vi "Grafica all plots.vi"(0 "prova":i32, 1 "ID COLLEGAMENTI":i32[](array[numeric]), 2 "Array scelte grafici":refnum<vi>[](array[refnum]), 3 "Array Grafici":refnum<vi>[](array[refnum]), 4 "array interpolazioni":refnum<vi>[](array[refnum]), 5 "Collaudi di confronto":T3[](array[typedef]), 6 "Array plot":T2[](array[typedef]) {"PLOT"."GRANDEZZA Y" items=["Banco", "Anno", "Numero", "N° tabella", "Misura", "Tipo prova", "Progressivo Acq", "tempo[h:m:s]", "tempo acq[min]", "f [Hz]", "Uav [V]", "Iav [A]", "Tq [Nm]", "n [rpm]", "P1 [kW]", "P1 n[kW]", "Q [m3/h]", "Q n[m3/h]", "Q [l/min]", "Q n[l/min]", "H1 [m]", "Dislivello [m]", "Hdinamica [m]", "HvAsp [m]", "HvMand [m]", "HvTot [m]", "H2 [m]", "Htot [m]", "Htot n[m]", "P3 (Phyd) [kW]", "P3 (Phyd) n[kW]", "P2 [kW]", "P2 n[kW]", "P2 n ps[kW]", "eta motore [%]", "eta pompa [%]", "eta pompa n[%]", "eta gruppo [%]", "eta gruppo n[%]", "T acqua [°C]", "Densità liquido [kg/m3]", "P barometrica [mbar]", "pf", "Uch1 [V]", "Uch2 [V]", "Uch3 [V]", "Ich1 [A]", "Ich2 [A]", "Ich3 [A]", "Temp.amb[°C]", "Ru-w [ohm]", "DTavvolg. [°C]", "Tamb Freddo [°C]", "Ru-w Freddo [ohm]", "Tc1[°C]", "Tc2[°C]", "Tc3[°C]", "Tc4[°C]", "Tc5", "Tc6", "Tc7", "Tc8", "H1[Bar]", "H2[bar]", "P premist.[Bar]", "Pserb[bar]", "n°NPSH", "NPSH", "Htot Ref[m]", "NPSH_%caduta", "%caduta", "Qref [m3/h]", "MEI"]; "PLOT"."GRANDEZZA X" items=["Banco", "Anno", "Numero", "N° tabella", "Misura", "Tipo prova", "Progressivo Acq", "tempo[h:m:s]", "tempo acq[min]", "f [Hz]", "Uav [V]", "Iav [A]", "Tq [Nm]", "n [rpm]", "P1 [kW]", "P1 n[kW]", "Q [m3/h]", "Q n[m3/h]", "Q [l/min]", "Q n[l/min]", "H1 [m]", "Dislivello [m]", "Hdinamica [m]", "HvAsp [m]", "HvMand [m]", "HvTot [m]", "H2 [m]", "Htot [m]", "Htot n[m]", "P3 (Phyd) [kW]", "P3 (Phyd) n[kW]", "P2 [kW]", "P2 n[kW]", "P2 n ps[kW]", "eta motore [%]", "eta pompa [%]", "eta pompa n[%]", "eta gruppo [%]", "eta gruppo n[%]", "T acqua [°C]", "Densità liquido [kg/m3]", "P barometrica [mbar]", "pf", "Uch1 [V]", "Uch2 [V]", "Uch3 [V]", "Ich1 [A]", "Ich2 [A]", "Ich3 [A]", "Temp.amb[°C]", "Ru-w [ohm]", "DTavvolg. [°C]", "Tamb Freddo [°C]", "Ru-w Freddo [ohm]", "Tc1[°C]", "Tc2[°C]", "Tc3[°C]", "Tc4[°C]", "Tc5", "Tc6", "Tc7", "Tc8", "H1[Bar]", "H2[bar]", "P premist.[Bar]", "Pserb[bar]", "n°NPSH", "NPSH", "Htot Ref[m]", "NPSH_%caduta", "%caduta", "Qref [m3/h]", "MEI"]; "Assi grafico"."ASSE X" items=["X 1", "X 2"]; "Assi grafico"."ASSE Y" items=["Y 1", "Y 2", "Y 3", "Y 4"]}, 7 "Dati collaudo in corso":T3, 8 "Tabella in corso":i32, 9 "grafico generico":cluster{"X":i32, "Y":i32, "nome plot":string}, 10 "Grafici":T1[](array[typedef]) {"ASSE Y 5"."Decimali" min=0 max=6; "ASSE Y 4"."Decimali" min=0 max=6; "ASSE Y 3"."Decimali" min=0 max=6; "ASSE Y 2"."Decimali" min=0 max=6; "ASSE Y 1"."Decimali" min=0 max=6; "ASSE X 2"."Decimali" min=0 max=6; "ASSE X 1"."Decimali" min=0 max=6}, 11 "Legend:Autosize":bool) -> ()   [LabVIEW 2019]
uses:
  TypeDef/Dati collaudo.ctl
  TypeDef/Definizione_plot.ctl
  TypeDef/Definizione_Grafico_REPORT.ctl
panel:
  out "Array AND":bool[](array[boolean])
  out "Array Prova Resistenza":bool[](array[boolean])
  out "Nomi Grafici":string[](array[string])
  out "x-y":u32
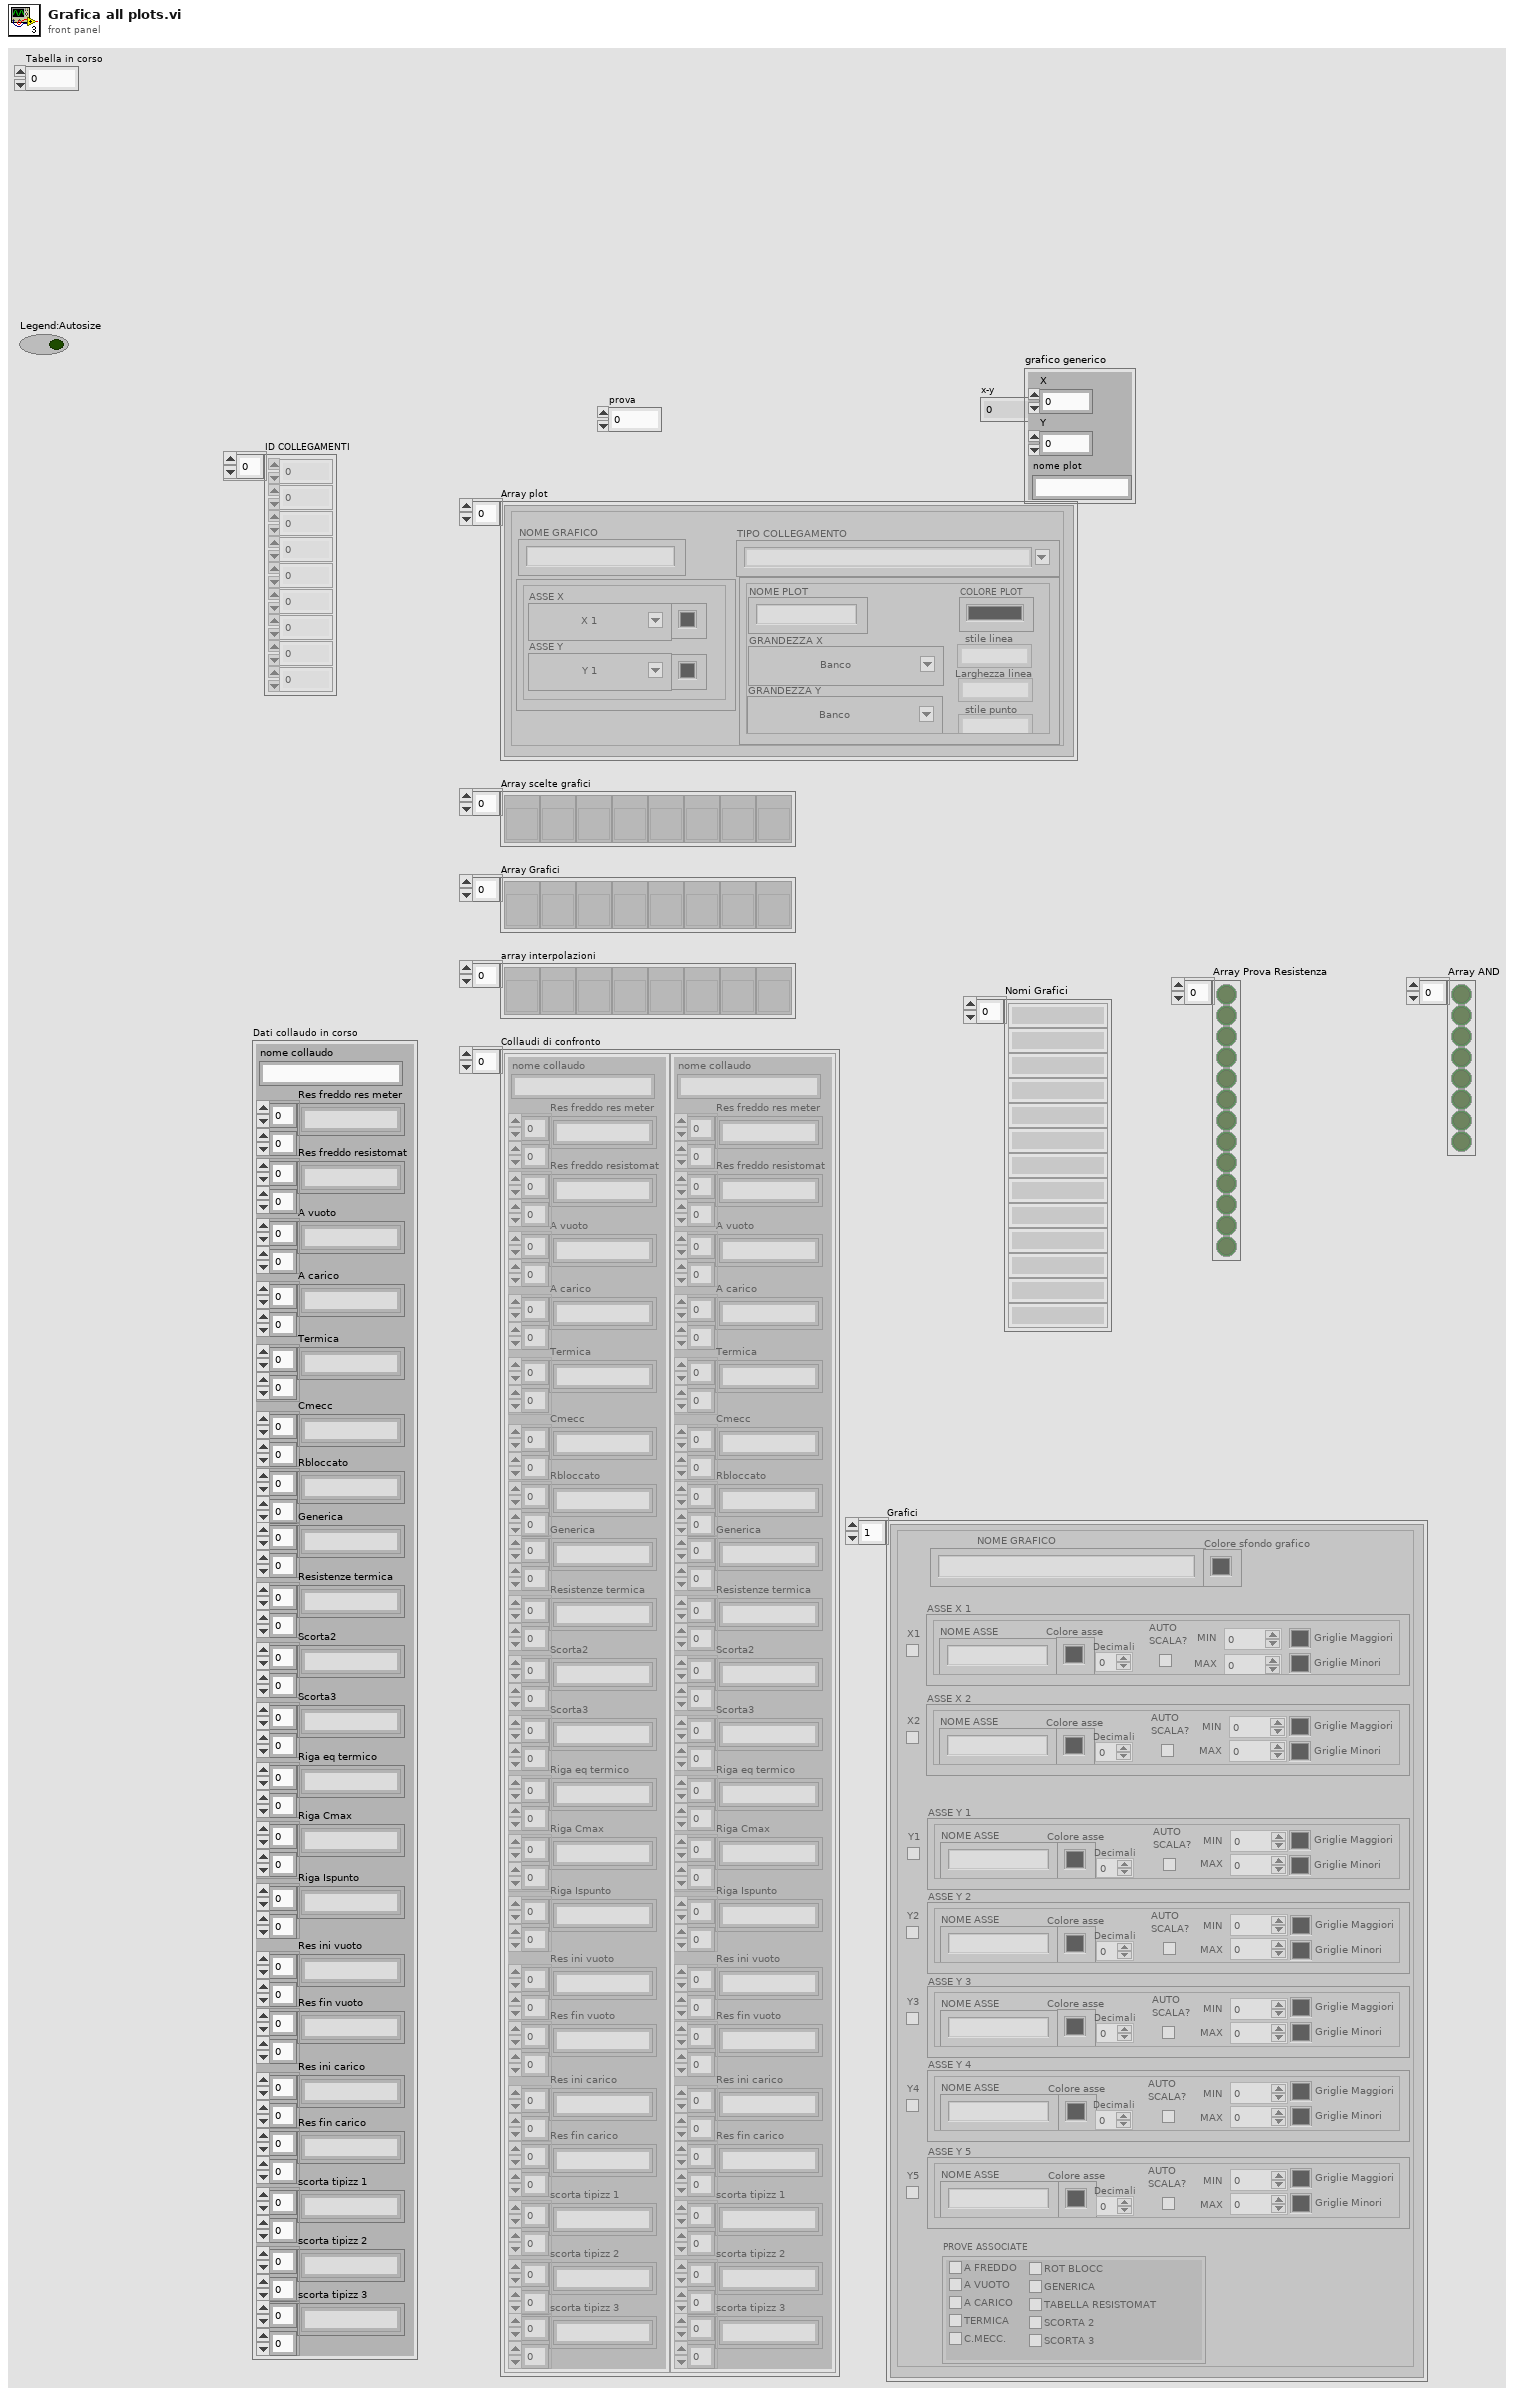
[diagram p1: front panel]
types:
  T1 = typedef "Definizione_Grafico_REPORT.ctl" = cluster{"ASSE X 1":cluster{"NOME ASSE":string, "AUTO\nSCALA?":bool, "MIN":dbl, "MAX":dbl, "Colore asse":u32, "Griglie Maggiori":u32, "Griglie Minori":u32, "Decimali":i8}, "ASSE X 2":cluster{"NOME ASSE":string, "AUTO\nSCALA?":bool, "MIN":dbl, "MAX":dbl, "Colore asse":u32, "Griglie Maggiori":u32, "Griglie Minori":u32, "Decimali":i8}, "ASSE Y 1":cluster{"NOME ASSE":string, "AUTO\nSCALA?":bool, "MIN":dbl, "MAX":dbl, "Colore asse":u32, "Griglie Maggiori":u32, "Griglie Minori":u32, "Decimali":i8}, "ASSE Y 2":cluster{"NOME ASSE":string, "AUTO\nSCALA?":bool, "MIN":dbl, "MAX":dbl, "Colore asse":u32, "Griglie Maggiori":u32, "Griglie Minori":u32, "Decimali":i8}, "ASSE Y 3":cluster{"NOME ASSE":string, "AUTO\nSCALA?":bool, "MIN":dbl, "MAX":dbl, "Colore asse":u32, "Griglie Maggiori":u32, "Griglie Minori":u32, "Decimali":i8}, "ASSE Y 4":cluster{"NOME ASSE":string, "AUTO\nSCALA?":bool, "MIN":dbl, "MAX":dbl, "Colore asse":u32, "Griglie Maggiori":u32, "Griglie Minori":u32, "Decimali":i8}, "X1":bool, "X2":bool, "Y1":bool, "Y2":bool, "Y3":bool, "Y4":bool, "NOME GRAFICO":string, "PROVE ASSOCIATE":cluster{"A FREDDO":bool, "A VUOTO":bool, "A CARICO":bool, "TERMICA":bool, "C.MECC.":bool, "ROT BLOCC":bool, "GENERICA":bool, "TABELLA RESISTOMAT":bool, "SCORTA 2":bool, "SCORTA 3":bool}, "ASSE Y 5":cluster{"NOME ASSE":string, "AUTO\nSCALA?":bool, "MIN":dbl, "MAX":dbl, "Colore asse":u32, "Griglie Maggiori":u32, "Griglie Minori":u32, "Decimali":i8}, "Y5":bool, "Colore sfondo grafico":u32}
  T2 = typedef "Definizione_plot.ctl" = cluster{"Assi grafico":cluster{"ASSE Y":u16, "ASSE X":u16, "Colore x":u32, "Colore y":u32}, "TIPO COLLEGAMENTO":string, "PLOT":cluster{"GRANDEZZA X":u16, "GRANDEZZA Y":u16, "COLORE PLOT":u32, "NOME PLOT":string, "Larghezza linea":u16, "stile linea":u16, "stile punto":u16}, "NOME GRAFICO":string}
  T3 = typedef "Dati collaudo.ctl" = cluster{"nome collaudo":string, "Res freddo res meter":string[][], "Res freddo resistomat":string[][], "A vuoto":string[][], "A carico":string[][], "Termica":string[][], "Cmecc":string[][], "Rbloccato":string[][], "Generica":string[][], "Resistenze termica":string[][], "Scorta2":string[][], "Scorta3":string[][], "Riga eq termico":string[][], "Riga Cmax":string[][], "Riga Ispunto":string[][], "Res ini vuoto":string[][], "Res fin vuoto":string[][], "Res ini carico":string[][], "Res fin carico":string[][], "scorta tipizz 1":string[][], "scorta tipizz 2":string[][], "scorta tipizz 3":string[][]}
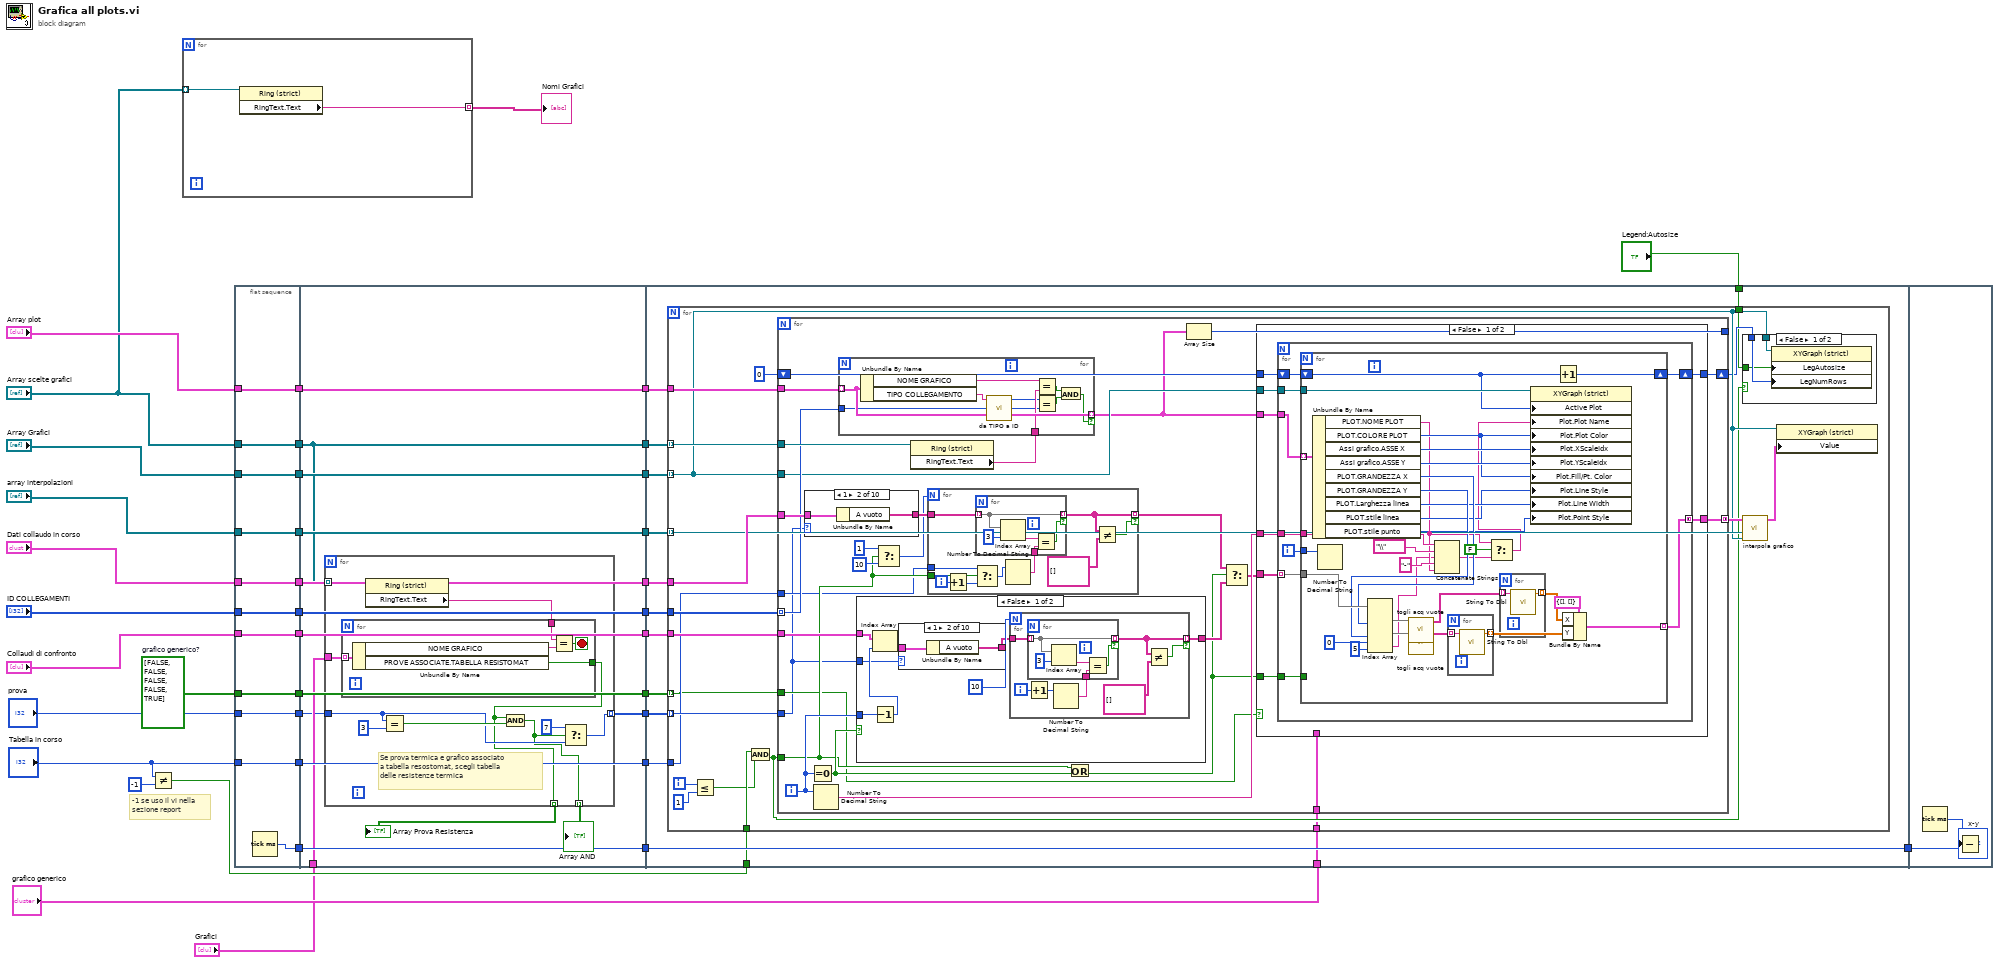
[diagram p0: block diagram]
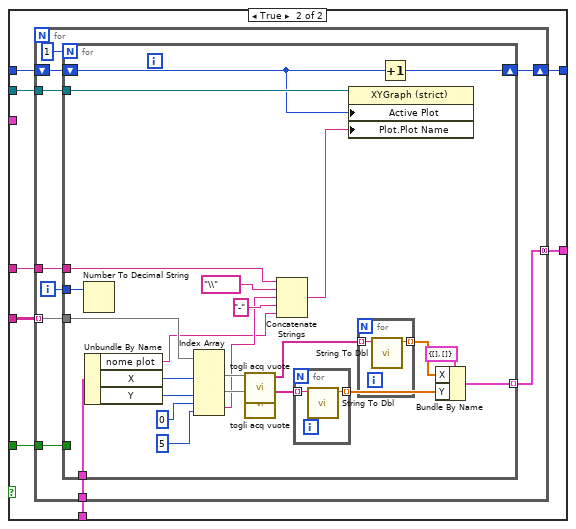
[diagram p3: hidden frame]
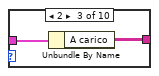
[diagram p5: hidden frame]
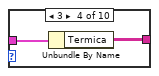
[diagram p6: hidden frame]
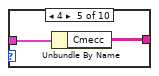
[diagram p7: hidden frame]
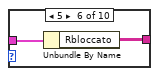
[diagram p8: hidden frame]
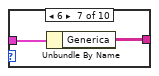
[diagram p9: hidden frame]
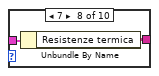
[diagram p10: hidden frame]
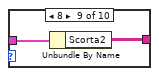
[diagram p11: hidden frame]
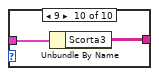
[diagram p12: hidden frame]
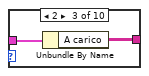
[diagram p14: hidden frame]
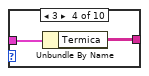
[diagram p15: hidden frame]
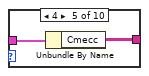
[diagram p16: hidden frame]
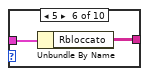
[diagram p17: hidden frame]
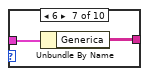
[diagram p18: hidden frame]
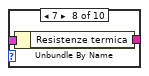
[diagram p19: hidden frame]
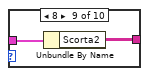
[diagram p20: hidden frame]
diagram:
  w6 = bool[] [FALSE, FALSE, FALSE, FALSE, TRUE]  # grafico generico?
  # "-1 se uso il vi nella\nsezione report"
  n1 = Not Equal?(x="Tabella in corso", y=-1) -> (x != y?=w29:bool)
  n2 = for {
    tunnel: "Array scelte grafici" -> [w41] mode=indexing
    tunnel: [w40] -> w2 mode=indexing
    n3 = property class="Ring (strict)"(reference=w41) -> ("RingText.Text"=w40:string)  [unwired: 1 in, 2 out]
  }
  "Nomi Grafici" <- w2
  n4 = flat-sequence {
    tunnel: "prova" -> [w45]
    tunnel: "Array scelte grafici" -> [w46]
    tunnel: "Array Grafici" -> [w47]
    tunnel: "Array plot" -> [w48]
    tunnel: "Dati collaudo in corso" -> [w49]
    tunnel: "Collaudi di confronto" -> [w50]
    tunnel: "ID COLLEGAMENTI" -> [w51]
    tunnel: "array interpolazioni" -> [w52]
    tunnel: [w52] -> w28
    tunnel: [w51] -> w26
    tunnel: [w50] -> w24
    tunnel: [w49] -> w22
    tunnel: [w48] -> w20
    tunnel: [w47] -> w18
    tunnel: [w46] -> w16
    tunnel: [w45] -> w14
    tunnel: [w44] -> w12
    tunnel: "Tabella in corso" -> [w43]
    tunnel: [w43] -> w10
    tunnel: [w42] -> w7
    tunnel: w6 -> [w42]
    tunnel: w28 -> [w67]
    tunnel: [w67] -> w27
    tunnel: w26 -> [w66]
    tunnel: [w66] -> w25
    tunnel: w24 -> [w65]
    tunnel: [w65] -> w23
    tunnel: w22 -> [w64]
    tunnel: [w64] -> w21
    tunnel: w20 -> [w63]
    tunnel: [w63] -> w19
    tunnel: w18 -> [w60]
    tunnel: [w60] -> w17
    tunnel: w16 -> [w57]
    tunnel: [w57] -> w15
    tunnel: w14 -> [w56]
    tunnel: [w55] -> w13
    tunnel: w12 -> [w62]
    tunnel: [w62] -> w11
    tunnel: w10 -> [w61]
    tunnel: [w61] -> w9
    tunnel: [w59] -> w8
    tunnel: w7 -> [w59]
    tunnel: "Grafici" -> [w58]
    tunnel: w27 -> [w96]
    tunnel: w25 -> [w95]
    tunnel: w23 -> [w94]
    tunnel: w21 -> [w93]
    tunnel: w19 -> [w92]
    tunnel: w17 -> [w91]
    tunnel: w15 -> [w90]
    tunnel: w13 -> [w89]
    tunnel: w11 -> [w88]
    tunnel: [w88] -> w32
    tunnel: w9 -> [w87]
    tunnel: w29 -> [w86]
    tunnel: w8 -> [w85]
    tunnel: "grafico generico" -> [w84]
    tunnel: "Legend:Autosize" -> [w83]
    tunnel: w32 -> [w329]
    frame #0 {
      n5 = Tick Count (ms)() -> (millisecond timer value=w44:u32)
    }
    frame #1 {
      n6 = for {
        tunnel: w58 -> [w77]
        tunnel: w57 -> [w76] mode=indexing
        tunnel: w56 -> [w72]
        tunnel: [w71] -> w55 mode=indexing
        tunnel: [w69] -> w54 mode=indexing
        tunnel: [w68] -> w53 mode=indexing
        # "Se prova termica e grafico associato\na tabella resostomat, scegli tabella \ndelle resistenze termica"
        n7 = property class="Ring (strict)"(reference=w76) -> ("RingText.Text"=w75:string)  [unwired: 1 in, 2 out]
        n8 = for {
          tunnel: w77 -> [w82] mode=indexing
          tunnel: w75 -> [w80]
          tunnel: [w78] -> w69
          stop <- w79 stop-if-true
          n9 = Unbundle By Name(w82) -> ("NOME GRAFICO"=w81:string, "PROVE ASSOCIATE.TABELLA RESISTOMAT"=w78:bool)
          n10 = Equal?(x=w80, y=w81) -> (x = y?=w79:bool)
        }
        n11 = Equal?(x=w72, y=3) -> (x = y?=w73:bool)
        n12 = And(x=w69, y=w73) -> (x .and. y?=w68:bool)
        n13 = Select(t=7, s=w68, f=w72) -> (s? t:f=w71:i32)
      }
      "Array Prova Resistenza" <- w54
      "Array AND" <- w53
    }
    frame #2 {
      n14 = for {
        tunnel: w90 -> [w113] mode=indexing
        tunnel: w91 -> [w107] mode=indexing
        tunnel: w92 -> [w117]
        tunnel: w93 -> [w116]
        tunnel: w94 -> [w115]
        tunnel: w95 -> [w114]
        tunnel: w96 -> [w110] mode=indexing
        tunnel: w89 -> [w109] mode=indexing
        tunnel: w87 -> [w104]
        tunnel: w86 -> [w103]
        tunnel: w85 -> [w99] mode=indexing
        tunnel: w84 -> [w98]
        tunnel: w83 -> [w97]
        i -> [w106]
        n15 = Less Or Equal?(x=w106, y=1) -> (x <= y?=w102:bool)
        n16 = And(x=w103, y=w102) -> (x .and. y?=w101:bool)
        n17 = for {
          tunnel: w117 -> [w147]
          tunnel: w113 -> [w146]
          tunnel: w107 -> [w141]
          tunnel: w116 -> [w145]
          tunnel: w115 -> [w135]
          tunnel: w114 -> [w144] mode=indexing
          tunnel: [w140] -> w112 mode=concatenating
          shift-right: [w139] -> w100
          shift-left: 0 -> [w138]
          tunnel: w109 -> [w121]
          tunnel: [w130] -> _
          tunnel: w101 -> [w126]
          tunnel: w104 -> [w125]
          tunnel: w99 -> [w123]
          tunnel: w98 -> [w122]
          i -> [w134]
          n18 = case shown="1" w121 {
            tunnel: w145 -> [_ w249 w251 w253 w255 w257 w259 w261 w263 w265]
            tunnel: [_ w248 w250 w252 w254 w256 w258 w260 w262 w264] -> w143
            frame 0, Default {
            }
            frame 1 {
              n19 = Unbundle By Name(w249) -> ("A vuoto"=w248:string[][])
            }
            frame 2 {
              n20 = Unbundle By Name(w251) -> ("A carico"=w250:string[][])
            }
            frame 3 {
              n21 = Unbundle By Name(w253) -> ("Termica"=w252:string[][])
            }
            frame 4 {
              n22 = Unbundle By Name(w255) -> ("Cmecc"=w254:string[][])
            }
            frame 5 {
              n23 = Unbundle By Name(w257) -> ("Rbloccato"=w256:string[][])
            }
            frame 6 {
              n24 = Unbundle By Name(w259) -> ("Generica"=w258:string[][])
            }
            frame 7 {
              n25 = Unbundle By Name(w261) -> ("Resistenze termica"=w260:string[][])
            }
            frame 8 {
              n26 = Unbundle By Name(w263) -> ("Scorta2"=w262:string[][])
            }
            frame 9 {
              n27 = Unbundle By Name(w265) -> ("Scorta3"=w264:string[][])
            }
          }
          n28 = Equal To 0?(x=w134) -> (x = 0?=w133:bool)
          n29 = Number To Decimal String(number=w134) -> (decimal integer string=w142:string)  [unwired: 1 in]
          n30 = case shown="False" w133 {
            tunnel: w135 -> [w272 _]
            tunnel: w134 -> [w271 _]
            tunnel: [w269 _] -> w132
            tunnel: w121 -> [w266 _]
            frame False {
              n31 = Decrement(x=w271) -> (x-1=w270:i32)
              n32 = Index Array(array=w272, index=w270) -> (element=w268:T3)
              n33 = case shown="1" w266 {
                tunnel: w268 -> [_ w275 w277 w279 w281 w283 w285 w287 w289 w291]
                tunnel: [_ w274 w276 w278 w280 w282 w284 w286 w288 w290] -> w267
                frame 0, Default {
                }
                frame 1 {
                  n34 = Unbundle By Name(w275) -> ("A vuoto"=w274:string[][])
                }
                frame 2 {
                  n35 = Unbundle By Name(w277) -> ("A carico"=w276:string[][])
                }
                frame 3 {
                  n36 = Unbundle By Name(w279) -> ("Termica"=w278:string[][])
                }
                frame 4 {
                  n37 = Unbundle By Name(w281) -> ("Cmecc"=w280:string[][])
                }
                frame 5 {
                  n38 = Unbundle By Name(w283) -> ("Rbloccato"=w282:string[][])
                }
                frame 6 {
                  n39 = Unbundle By Name(w285) -> ("Generica"=w284:string[][])
                }
                frame 7 {
                  n40 = Unbundle By Name(w287) -> ("Resistenze termica"=w286:string[][])
                }
                frame 8 {
                  n41 = Unbundle By Name(w289) -> ("Scorta2"=w288:string[][])
                }
                frame 9 {
                  n42 = Unbundle By Name(w291) -> ("Scorta3"=w290:string[][])
                }
              }
              n43 = for {
                N: 10 -> [_]
                tunnel: w267 -> [w296]
                tunnel: [w293] -> w269 mode=indexing if=w292
                i -> [w298]
                n44 = Increment(x=w298) -> (x+1=w297:i32)
                n45 = Number To Decimal String(number=w297) -> (decimal integer string=w295:string)  [unwired: 1 in]
                n46 = for {
                  tunnel: w296 -> [w303] mode=indexing
                  tunnel: [w303] -> w293 mode=indexing if=w300
                  tunnel: w295 -> [w301]
                  n47 = Index Array(array=w303, index=3) -> (element=w302:string)
                  n48 = Equal?(x=w302, y=w301) -> (x = y?=w300:bool)
                }
                n49 = Not Equal?(x=w293, y=string[][] [] ("Scorta3")) -> (x != y?=w292:bool)
              }
            }
            frame True {
            }
          }
          n50 = Select(t=1, s=w126, f=10) -> (s? t:f=w127:i32)
          n51 = property class="Ring (strict)"(reference=w146) -> ("RingText.Text"=w148:string)  [unwired: 1 in, 2 out]
          n52 = for {
            tunnel: w147 -> [w327] mode=indexing
            tunnel: w148 -> [w325]
            tunnel: [w327] -> w131 mode=indexing if=w321
            tunnel: w144 -> [w324]
            n53 = Unbundle By Name(w327) -> ("NOME GRAFICO"=w326:string, "TIPO COLLEGAMENTO"=w320:string)
            n54 = call "da TIPO a ID.vi"("TIPO"=w320) -> ("ID"=w319:i32)  [unwired: 10 in]
            n55 = Equal?(x=w326, y=w325) -> (x = y?=w323:bool)
            n56 = Equal?(x=w319, y=w324) -> (x = y?=w322:bool)
            n57 = And(x=w323, y=w322) -> (x .and. y?=w321:bool)
          }
          n58 = for {
            N: w127 -> [_]
            tunnel: w143 -> [w312]
            tunnel: [w309] -> w137 mode=indexing if=w308
            tunnel: w126 -> [w307]
            tunnel: w125 -> [w304]
            i -> [w313]
            n59 = Increment(x=w313) -> (x+1=w306:i32)
            n60 = Select(t=w304, s=w307, f=w306) -> (s? t:f=w305:i32)
            n61 = Number To Decimal String(number=w305) -> (decimal integer string=w311:string)  [unwired: 1 in]
            n62 = for {
              tunnel: w312 -> [w318] mode=indexing
              tunnel: [w318] -> w309 mode=indexing if=w315
              tunnel: w311 -> [w316]
              n63 = Index Array(array=w318, index=3) -> (element=w317:string)
              n64 = Equal?(x=w317, y=w316) -> (x = y?=w315:bool)
            }
            n65 = Not Equal?(x=w309, y=string[][] [] ("Scorta3")) -> (x != y?=w308:bool)
          }
          n66 = Or(x=w126, y=w133) -> (x .or. y?=w124:bool)
          n67 = Array Size(array=w131) -> (size(s)=w130:i32)
          n68 = Select(t=w137, s=w124, f=w132) -> (s? t:f=w136:string[][][])
          n69 = case shown="False" w123 {
            tunnel: w142 -> [w156 w209]
            tunnel: w141 -> [w155 w208]
            tunnel: [w154 w207] -> w140
            tunnel: [w153 w206] -> w139
            tunnel: w138 -> [w152 w205]
            tunnel: w136 -> [w151 w204]
            tunnel: w131 -> [w150 _]
            tunnel: w124 -> [w149 w203]
            tunnel: w122 -> [_ w202]
            frame False {
              n70 = for {
                tunnel: w155 -> [w165]
                tunnel: w150 -> [w164]
                tunnel: w151 -> [w163] mode=indexing
                tunnel: w156 -> [w161]
                shift-right: [w159] -> w153
                shift-left: w152 -> [w160]
                tunnel: [w158] -> w154 mode=concatenating
                tunnel: w149 -> [w157]
                i -> [w162]
                n71 = for {
                  tunnel: w165 -> [w196]
                  tunnel: w164 -> [w197] mode=indexing
                  tunnel: w163 -> [w189]
                  tunnel: w162 -> [w192]
                  tunnel: w161 -> [w190]
                  shift-right: [w188] -> w159
                  shift-left: w160 -> [w187]
                  tunnel: [w177] -> w158 mode=indexing
                  tunnel: w157 -> [_]
                  n72 = Unbundle By Name(w197) -> ("PLOT.NOME PLOT"=w172:string, "PLOT.COLORE PLOT"=w176:u32, "Assi grafico.ASSE X"=w195:u16, "Assi grafico.ASSE Y"=w194:u16, "PLOT.GRANDEZZA X"=w186:u16, "PLOT.GRANDEZZA Y"=w185:u16, "PLOT.Larghezza linea"=w175:u16, "PLOT.stile linea"=w174:u16, "PLOT.stile punto"=w173:u16)
                  n73 = Number To Decimal String(number=w192) -> ()  [unwired: 1 in, 1 out]
                  n74 = Index Array(array=w189, index (col) #1=w186, index (col) #2=w185, index (row) #3=0 ("disabled index (row)"), index (col) #3=5 ("disabled index (col)")) -> (element #1=w183:string[], element #2=w182:string[], element #3=w166:string)  [unwired: 2 in]
                  n75 = call "togli acq vuote.vi"("Q"=w183) -> ("Array"=w181:string[])  [unwired: 10 in]
                  n76 = call "togli acq vuote.vi"("Q"=w182) -> ("Array"=w179:string[])  [unwired: 10 in]
                  n77 = Concatenate Strings(w190, "\\" ("string"), w166, "-" ("string"), w172) -> (w171:string)
                  n78 = for {
                    tunnel: w179 -> [w199] mode=indexing
                    tunnel: [w198] -> w178 mode=indexing
                    n79 = call "String To Dbl.vi"("String"=w199) -> ("Numeric"=w198:dbl)  [unwired: 10 in]
                  }
                  n80 = Select(t=w172, s=FALSE, f=w171) -> (s? t:f=w170:string)
                  n81 = for {
                    tunnel: w181 -> [w201] mode=indexing
                    tunnel: [w200] -> w180 mode=indexing
                    n82 = call "String To Dbl.vi"("String"=w201) -> ("Numeric"=w200:dbl)  [unwired: 10 in]
                  }
                  n83 = property class="XYGraph (strict)"(reference=w196, "Active Plot"=w187, "Plot.Plot Name"=w170, "Plot.Plot Color"=w176, "Plot.XScaleIdx"=w195, "Plot.YScaleIdx"=w194, "Plot.Fill/Pt. Color"=w176, "Plot.Line Style"=w174, "Plot.Line Width"=w175, "Plot.Point Style"=w173) -> ()  [unwired: 1 in, 2 out]
                  n84 = Increment(x=w187) -> (x+1=w188:i32)
                  n85 = Bundle By Name(cluster=cluster{"X":dbl[], "Y":dbl[]} {"X"=[], "Y"=[]}, "X"=w180, "Y"=w178) -> (w177:cluster{"X":dbl[], "Y":dbl[]})
                }
              }
            }
            frame True {
              n86 = for {
                tunnel: w208 -> [w219]
                tunnel: w204 -> [w218] mode=indexing
                tunnel: w209 -> [w216]
                shift-right: [w214] -> w206
                shift-left: w205 -> [w215]
                tunnel: [w213] -> w207 mode=concatenating
                tunnel: w203 -> [w212]
                tunnel: w202 -> [w211]
                i -> [w217]
                n87 = for {
                  N: 1 -> [_]
                  tunnel: w219 -> [w243]
                  tunnel: w218 -> [w238]
                  tunnel: w217 -> [w241]
                  tunnel: w216 -> [w239]
                  shift-right: [w237] -> w214
                  shift-left: w215 -> [w236]
                  tunnel: [w228] -> w213 mode=indexing
                  tunnel: w212 -> [_]
                  tunnel: w211 -> [w221]
                  n88 = Number To Decimal String(number=w241) -> ()  [unwired: 1 in, 1 out]
                  n89 = Unbundle By Name(w221) -> ("nome plot"=w220:string, "X"=w224:i32, "Y"=w223:i32)
                  n90 = Index Array(array=w238, index (col) #1=w224, index (col) #2=w223, index (row) #3=0 ("disabled index (row)"), index (col) #3=5 ("disabled index (col)")) -> (element #1=w234:string[], element #2=w233:string[], element #3=w225:string)  [unwired: 2 in]
                  n91 = call "togli acq vuote.vi"("Q"=w234) -> ("Array"=w232:string[])  [unwired: 10 in]
                  n92 = call "togli acq vuote.vi"("Q"=w233) -> ("Array"=w230:string[])  [unwired: 10 in]
                  n93 = Concatenate Strings(w239, "\\" ("string"), w225, "-" ("string"), w220) -> (w222:string)
                  n94 = for {
                    tunnel: w230 -> [w245] mode=indexing
                    tunnel: [w244] -> w229 mode=indexing
                    n95 = call "String To Dbl.vi"("String"=w245) -> ("Numeric"=w244:dbl)  [unwired: 10 in]
                  }
                  n96 = property class="XYGraph (strict)"(reference=w243, "Active Plot"=w236, "Plot.Plot Name"=w222) -> ()  [unwired: 1 in, 2 out]
                  n97 = for {
                    tunnel: w232 -> [w247] mode=indexing
                    tunnel: [w246] -> w231 mode=indexing
                    n98 = call "String To Dbl.vi"("String"=w247) -> ("Numeric"=w246:dbl)  [unwired: 10 in]
                  }
                  n99 = Increment(x=w236) -> (x+1=w237:i32)
                  n100 = Bundle By Name(cluster=cluster{"X":dbl[], "Y":dbl[]} {"X"=[], "Y"=[]}, "X"=w231, "Y"=w229) -> (w228:cluster{"X":dbl[], "Y":dbl[]})
                }
              }
            }
          }
        }
        n101 = case shown="False" w101 {
          tunnel: w107 -> [w120 _]
          tunnel: w100 -> [w119 _]
          tunnel: w97 -> [w118 _]
          frame False {
            n102 = property class="XYGraph (strict)"(reference=w120, "LegAutosize"=w118, "LegNumRows"=w119) -> ()  [unwired: 1 in, 2 out]
          }
          frame True {
          }
        }
        n103 = call "interpola grafico.vi"("graph ref"=w107, "Interpola"=w110, "Array"=w112) -> ("Array out"=w108:cluster{"X":dbl[], "Y":dbl[]}[])  [unwired: 8 in]
        n104 = property class="XYGraph (strict)"(reference=w107, "Value"=w108) -> ()  [unwired: 1 in, 2 out]
      }
    }
    frame #3 {
      n105 = Tick Count (ms)() -> (millisecond timer value=w330:u32)
      n106 = Subtract(x=w330, y=w329) -> (x-y=→"x-y":u32)
    }
  }
